vi "R&S HMP-4000 Heater.vi"() -> ()   [LabVIEW 2018]
panel:
  in  "Output State (Off)":bool
  out "CURRENT":dbl caption="Current Value" format="%.3f"
  out "VOLTAGE":dbl caption="Voltage Value" format="%.3f"
  in  "Voltage (0.0)":dbl format="%.3f"
  in  "Current (0.0)":dbl format="%.3f"
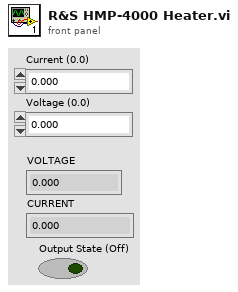
[diagram p1: front panel]
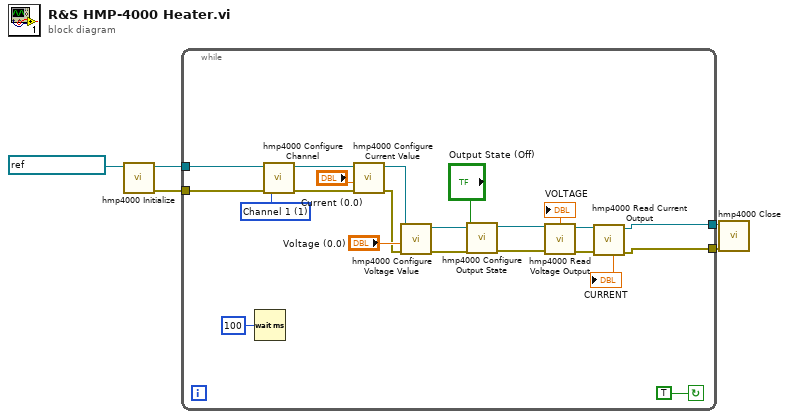
[diagram p0: block diagram]
diagram:
  n1 = call <instrlib>:"hmp4000 Initialize.vi"("VISA resource name"=refnum<visa-resource-name> "RS-HMP4000") -> ("error out"=w3:errorcluster, "VISA resource name out"=w4:refnum<visa-resource-name>)  [unwired: 9 in]
  n2 = while {
    tunnel: w4 -> [w27]
    tunnel: w3 -> [w26]
    tunnel: [w16] -> w2
    tunnel: [w15] -> w1
    stop <- TRUE continue-if-true
    w25 = 1 items=["Channel 1"=1, "Channel 2"=2, "Channel 3"=3, "Channel 4"=4] ("Channel (Channel 1)")
    n3 = Wait (ms)(milliseconds to wait=u32 100) -> ()  [unwired: 1 out]
    n4 = call <instrlib>:"hmp4000 Configure Channel.vi"("error in (no error)"=w26, "Channel (Channel 1)"=w25, "VISA resource name"=w27) -> ("error out"=w22:errorcluster, "VISA resource name out"=w24:refnum<visa-resource-name>)  [unwired: 7 in]
    n5 = call <instrlib>:"hmp4000 Configure Current Value.vi"("error in (no error)"=w22, "Current (0.0)"="Current (0.0)", "VISA resource name"=w24) -> ("error out"=w19:errorcluster, "VISA resource name out"=w23:refnum<visa-resource-name>)  [unwired: 7 in]
    n6 = call <instrlib>:"hmp4000 Configure Voltage Value.vi"("error in (no error)"=w19, "Voltage (0.0)"="Voltage (0.0)", "VISA resource name"=w23) -> ("error out"=w9:errorcluster, "VISA resource name out"=w10:refnum<visa-resource-name>)  [unwired: 7 in]
    n7 = call <instrlib>:"hmp4000 Configure Output State.vi"("error in (no error)"=w9, "Output State (Off)"="Output State (Off)", "VISA resource name"=w10) -> ("error out"=w7:errorcluster, "VISA resource name out"=w8:refnum<visa-resource-name>)  [unwired: 7 in]
    n8 = call <instrlib>:"hmp4000 Read Voltage Output.vi"("error in (no error)"=w7, "VISA resource name"=w8) -> ("error out"=w17:errorcluster, "Voltage Value"=→"VOLTAGE":dbl, "VISA resource name out"=w18:refnum<visa-resource-name>)  [unwired: 7 in]
    n9 = call <instrlib>:"hmp4000 Read Current Output.vi"("error in (no error)"=w17, "VISA resource name"=w18) -> ("error out"=w15:errorcluster, "Current Value"=→"CURRENT":dbl, "VISA resource name out"=w16:refnum<visa-resource-name>)  [unwired: 7 in]
  }
  n10 = call <instrlib>:"hmp4000 Close.vi"("error in (no error)"=w1, "VISA resource name"=w2) -> ()  [unwired: 9 in, 1 out]
